vi "ElevatorEncReset.vi"(11 "ElevEnc?":bool) -> ()   [LabVIEW 2017]
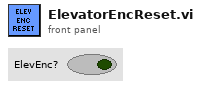
[diagram p1: front panel]
types:
  T1 = typedef "WPI_EncoderDevRef.ctl" = cluster{"DevStatus":errorcluster, "EncoderIndex":T2, "CounterIndex":T3, "DistancePerCount":dbl, "Decoding Type":T4}
  T2 = typedef "FPGA_EncoderIdx.ctl" = enum8{"Enc 0", "Enc 1", "Enc 2", "Enc 3", "Enc 4", "Enc 5", "Enc 6", "Enc 7", "Invalid"}
  T3 = typedef "FPGA_CounterCtrSystemIndex.ctl" = enum8{"Ctr 0", "Ctr 1", "Ctr 2", "Ctr 3", "Ctr 4", "Ctr 5", "Ctr 6", "Ctr 7", "Invalid"}
  T4 = typedef "WPI_EncoderType.ctl" = enum16{"1x", "2x", "4x"}
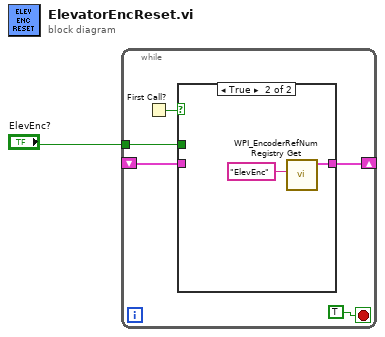
[diagram p0: block diagram]
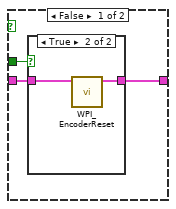
[diagram p2: hidden frame]
diagram:
  n1 = while {
    tunnel: "ElevEnc?" -> [w6]
    shift-right: [w5] -> _
    shift-left: _ -> [w4]
    stop <- TRUE stop-if-true
    n2 = First Call?() -> (First Call?: T/F=w3:bool)
    n3 = case shown="True" w3 {
      tunnel: w6 -> [w9 _]
      tunnel: [w7 w13] -> w5
      tunnel: w4 -> [w8 _]
      frame False {
        n4 = case shown="True" w9 {
          tunnel: [w10 w11] -> w7
          tunnel: w8 -> [w10 w12]
          frame False {
          }
          frame True {
            n5 = call <vilib>:"WPI_EncoderReset.vi"("EncoderDevRef"=w12) -> ("EncoderDevRef"=w11:T1)  [unwired: 9 in, 1 out]
          }
        }
      }
      frame True {
        n6 = call <vilib>:"WPI_EncoderRefNum Registry Get.vi"("refnum name"="ElevEnc") -> ("EncoderDevRef"=w13:T1)  [unwired: 9 in, 1 out]
      }
    }
  }
